vi "Read Coefficient Set.vi"(8 "error in (no error)":errorcluster, 10 "scale index":i32, 11 "Polynomial Scale configuration in":refnum<class "Polynomial Scale configuration.lvclass">) -> (0 "error out":errorcluster, 2 "Coefficients":dbl[](array[numeric]), 3 "Polynomial Scale configuration out":refnum<class "Polynomial Scale configuration.lvclass">)   [LabVIEW 2013, in "Polynomial Scale configuration.lvclass"]
uses:
  Polynomial Scale configuration.lvclass
  Polynomial Scale configuration.lvclass/Polynomial Scale configuration.ctl
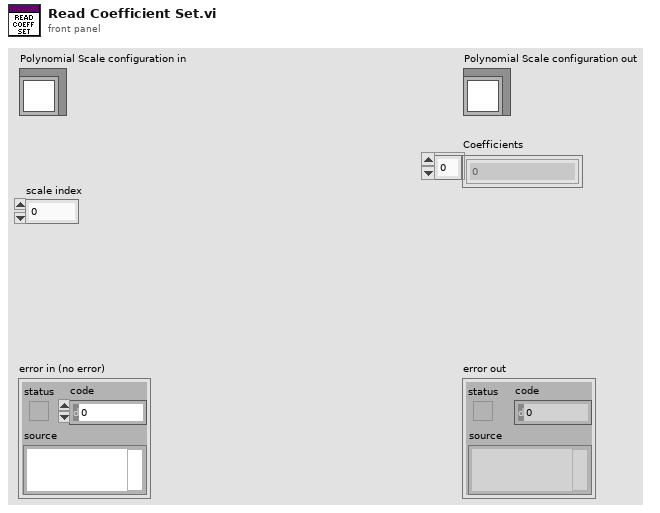
[diagram p1: front panel]
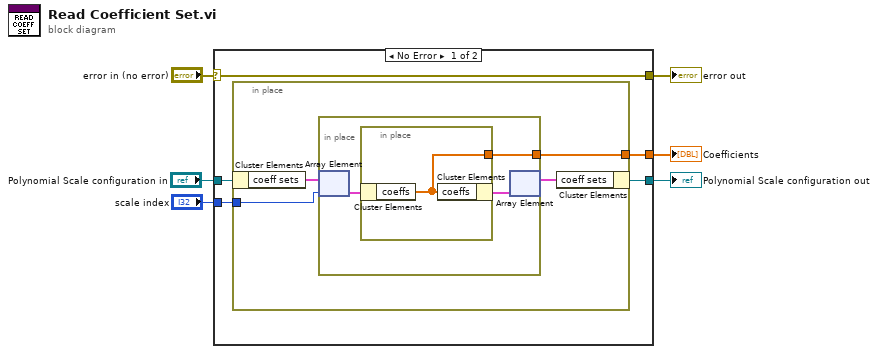
[diagram p0: block diagram]
diagram:
  n1 = case shown="No Error" "error in (no error)" {
    selector: "error in (no error)" -> [w11 w21]
    tunnel: [w11 w21] -> w5
    tunnel: [w8 w20] -> w3
    tunnel: "Polynomial Scale configuration in" -> [w10 w20]
    tunnel: "scale index" -> [w9 _]
    tunnel: [w7 _] -> w1
    frame No Error {
      n2 = in-place {
        in-place-border: w9 -> [w14]
        in-place-border: [w12] -> w7
        n3 = in-place-cluster #1(w10) -> ("coeff sets"=w15:cluster{"coeffs":dbl[]}[])
        n4 = in-place {
          in-place-border: [w16] -> w12
          n5 = in-place-array #2(w15, w14) -> (w18:cluster{"coeffs":dbl[]})
          n6 = in-place {
            in-place-border: [w19] -> w16
            n7 = in-place-cluster #3(w18) -> ("coeffs"=w19:dbl[])
            n8 = in-place-cluster #3("coeffs"=w19) -> (w17:cluster{"coeffs":dbl[]})
          }
          n9 = in-place-array #2(w17) -> (w13:cluster{"coeffs":dbl[]}[])  [unwired: 1 out]
        }
        n10 = in-place-cluster #1("coeff sets"=w13) -> (w8:refnum<class "Polynomial Scale configuration.lvclass">)
      }
    }
    frame Error {
    }
  }
  "error out" <- w5
  "Polynomial Scale configuration out" <- w3
  "Coefficients" <- w1
